vi "close underlying connection.vi"(8 "error in":errorcluster, 11 "connection in":refnum<class "connection maintainer.lvclass">) -> (0 "error out":errorcluster)   [LabVIEW 2015, in "connection maintainer.lvclass"]
uses:
  connection maintainer.lvclass
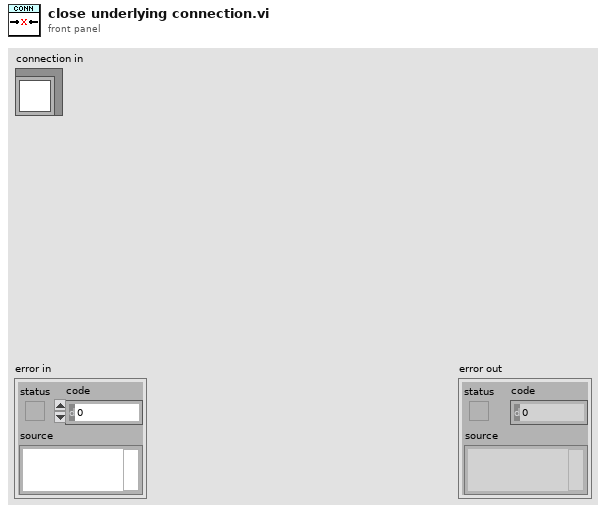
[diagram p1: front panel]
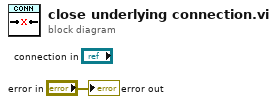
[diagram p0: block diagram]
diagram:
  "error out" <- "error in"
